vi "setPoint.vi"(8 "error in (no error)":errorcluster, 10 "point":T1, 11 "Waypoint in":refnum<class "Waypoint.lvclass">) -> (0 "error out":errorcluster, 3 "Waypoint out":refnum<class "Waypoint.lvclass">)   [LabVIEW 2009]
uses:
  Waypoint.lvclass
  point.ctl
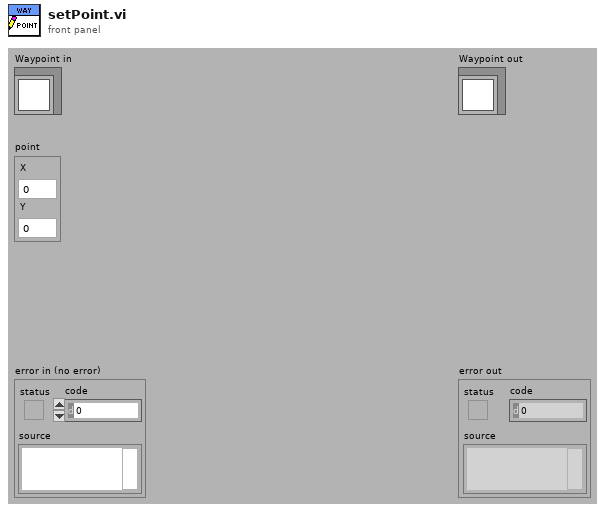
[diagram p1: front panel]
types:
  T1 = typedef "Waypoint.lvclass/point.ctl" = cluster{"X":dbl, "Y":dbl}
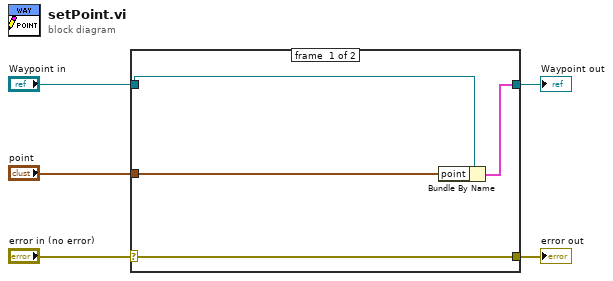
[diagram p0: block diagram]
diagram:
  n1 = case shown="No Error" "error in (no error)" {
    selector: "error in (no error)" -> [w9 w10]
    tunnel: [w9 w10] -> w4
    tunnel: [w7 w11] -> w2
    tunnel: "Waypoint in" -> [w8 w11]
    tunnel: "point" -> [w6 _]
    frame #0 {
      n2 = Bundle By Name(cluster=w8, "point"=w6) -> (w7:cluster{})
    }
    frame #1 {
    }
  }
  "error out" <- w4
  "Waypoint out" <- w2
